vi "PC_Main.vi"() -> ()   [LabVIEW 2018]
uses:
  Com/WebSockets/Data Def/Websocket Command.ctl
panel:
  out "x-y":u32
  out "Waveform Chart":T1(graph)
  in  "stop":bool
  out "Channel Size":i32
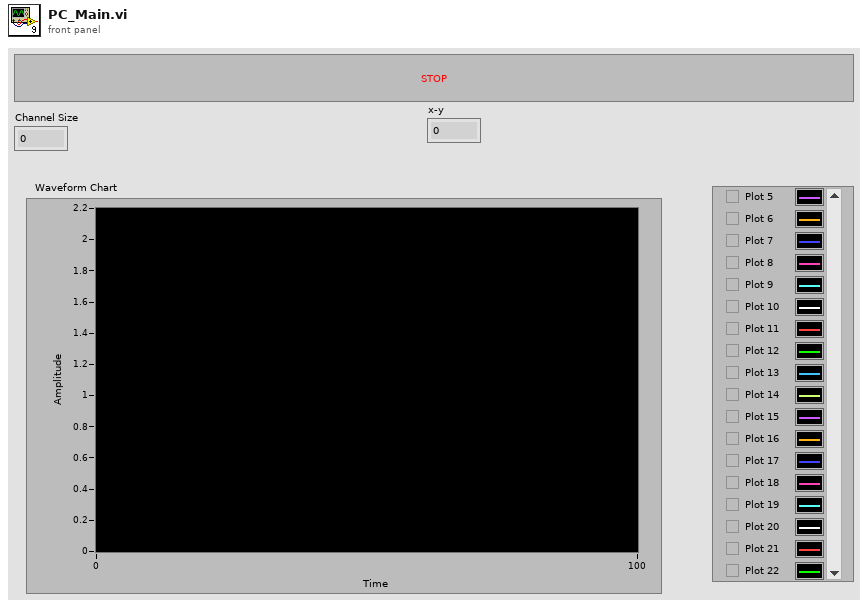
[diagram p1: front panel]
types:
  T1 = cluster{"[0]":dbl, "[1]":dbl, "[2]":dbl, "[3]":dbl, "[4]":dbl, "[5]":dbl, "[6]":dbl, "[7]":dbl, "[8]":dbl, "[9]":dbl, "[10]":dbl, "[11]":dbl, "[12]":dbl, "[13]":dbl, "[14]":dbl, "[15]":dbl, "[16]":dbl, "[17]":dbl, "[18]":dbl, "[19]":dbl, "[20]":dbl, "[21]":dbl, "[22]":dbl, "[23]":dbl, "[24]":dbl, "[25]":dbl, "[26]":dbl, "[27]":dbl, "[28]":dbl, "[29]":dbl, "[30]":dbl, "[31]":dbl, "[32]":dbl, "[33]":dbl, "[34]":dbl, "[35]":dbl, "[36]":dbl, "[37]":dbl, "[38]":dbl, "[39]":dbl, "[40]":dbl, "[41]":dbl, "[42]":dbl, "[43]":dbl, "[44]":dbl, "[45]":dbl, "[46]":dbl, "[47]":dbl, "[48]":dbl, "[49]":dbl, "[50]":dbl, "[51]":dbl, "[52]":dbl, "[53]":dbl, "[54]":dbl, "[55]":dbl, "[56]":dbl, "[57]":dbl, "[58]":dbl, "[59]":dbl, "[60]":dbl, "[61]":dbl, "[62]":dbl, "[63]":dbl, "[64]":dbl, "[65]":dbl, "[66]":dbl, "[67]":dbl, "[68]":dbl, "[69]":dbl, "[70]":dbl, "[71]":dbl, "[72]":dbl, "[73]":dbl, "[74]":dbl, "[75]":dbl, "[76]":dbl, "[77]":dbl, "[78]":dbl, "[79]":dbl, "[80]":dbl, "[81]":dbl, "[82]":dbl, "[83]":dbl, "[84]":dbl, "[85]":dbl, "[86]":dbl, "[87]":dbl, "[88]":dbl, "[89]":dbl, "[90]":dbl, "[91]":dbl, "[92]":dbl, "[93]":dbl, "[94]":dbl, "[95]":dbl}
  T2 = typedef "Websocket Command.ctl" = cluster{"Command":string, "Data":string}
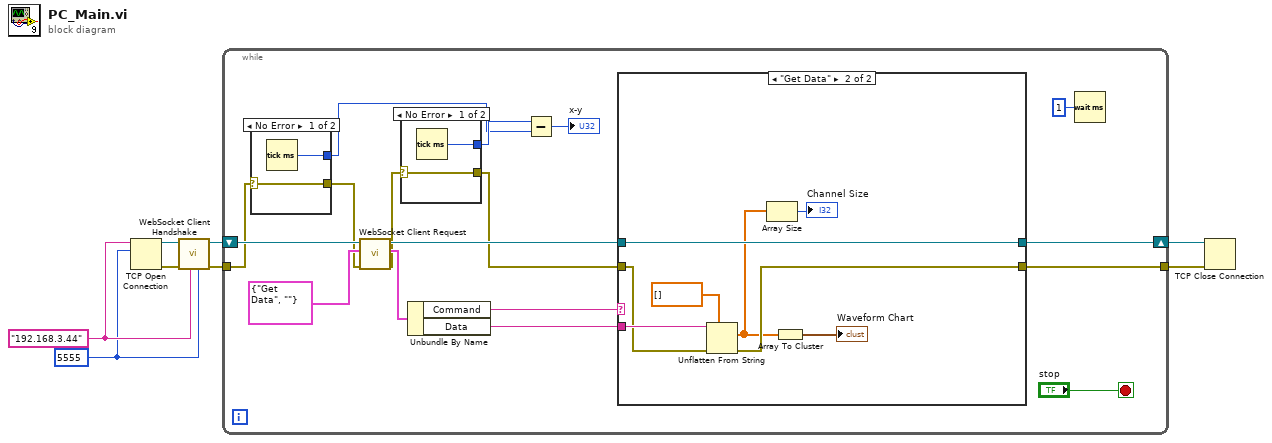
[diagram p0: block diagram]
diagram:
  w5 = u16 5555 ("remote port or service name")
  w6 = "192.168.3.44" ("address")
  n1 = TCP Open Connection(address=w6, remote port or service name=w5) -> (connection ID=w7:refnum<k5>, error out=w8:errorcluster)  [unwired: 3 in]
  n2 = call "WebSocket Client Handshake.vi"("remote port or service name"=w5, "address"=w6, "error in (no error)"=w8, "WebSocket Connection in"=w7) -> ("error out"=w4:errorcluster, "WebSocket Connection out"=w3:refnum<k5>)  [unwired: 5 in, 1 out]
  n3 = while {
    tunnel: w4 -> [w15]
    shift-right: [w18] -> w2
    shift-left: w3 -> [w25]
    tunnel: [w20] -> w1
    stop <- "stop" stop-if-true
    n4 = case shown="No Error" w15 {
      selector: w15 -> [w30 w31]
      tunnel: [w30 w31] -> w14
      tunnel: [w29 _] -> w10
      frame No Error {
        n5 = Tick Count (ms)() -> (millisecond timer value=w29:u32)
      }
      frame Error {
      }
    }
    n6 = call "WebSocket Client Request.vi"("error in"=w14, "Websocket Command In"=T2 {"Command"="Get Data", "Data"=""}, "WebSocket Connection in"=w25) -> ("error out"=w13:errorcluster, "Websocket Command Out"=w23:T2, "WebSocket Connection out"=w19:refnum<k5>)  [unwired: 6 in]
    n7 = case shown="No Error" w13 {
      selector: w13 -> [w27 w28]
      tunnel: [w27 w28] -> w12
      tunnel: [w26 _] -> w11
      frame No Error {
        n8 = Tick Count (ms)() -> (millisecond timer value=w26:u32)
      }
      frame Error {
      }
    }
    n9 = Unbundle By Name(w23) -> ("Command"=w22:string, "Data"=w21:string)
    n10 = Subtract(x=w11, y=w10) -> (x-y=→"x-y":u32)
    n11 = case shown="\"Get Data\"" w22 {
      tunnel: w12 -> [w33 w39]
      tunnel: w21 -> [_ w40]
      tunnel: [w33 w37] -> w20
      tunnel: w19 -> [w32 w41]
      tunnel: [w32 w41] -> w18
      frame Default {
      }
      frame "Get Data" {
        n12 = Unflatten From String(type=dbl[] [], binary string=w40, error in (no error)=w39) -> (value=w35:dbl[], error out=w37:errorcluster)  [unwired: 2 in, 1 out]
        n13 = Array Size(array=w35) -> (size(s)=→"Channel Size":i32)
        n14 = Array To Cluster(array=w35) -> (cluster=→"Waveform Chart":T1)
      }
    }
    n15 = Wait (ms)(milliseconds to wait=u32 1) -> ()  [unwired: 1 out]
  }
  n16 = TCP Close Connection(connection ID=w2, error in (no error)=w1) -> ()  [unwired: 1 in, 2 out]
